vi "PAM Volts per Bit.vi"() -> ()   [LabVIEW 2020, in "PAM Library.lvlib"]
uses:
  PAM Library.lvlib
panel:
  in  "Volts per Bit":dbl
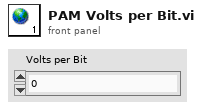
[diagram p1: front panel]
diagram:
